vi "Pockels-Initialise sequence for funct acq.vi"() -> (1 "Count towards trigger target (ms)":dbl format="%#_9g", 2 "Excess (us)":dbl format="%#_9g", 3 "waveform out":waveform(dbl)(graph))   [LabVIEW 2017]
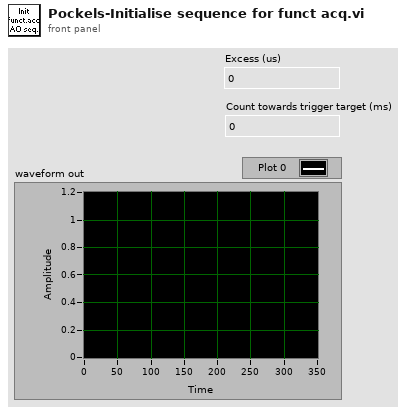
[diagram p1: front panel]
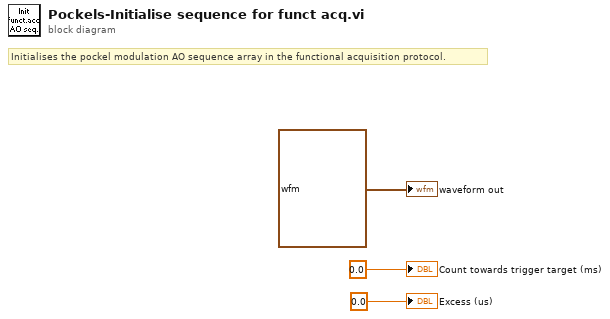
[diagram p0: block diagram]
diagram:
  # "Initialises the pockel modulation AO sequence array in the functional acquisition protocol."
  "waveform out" <- waveform(dbl) {"t0"=timestamp(0 s since 1904-01-01), "dt"=0.0, "Y"=[]} ("waveform out")
  "Excess (us)" <- 0.0 ("Count towards trigger target (us)")
  "Count towards trigger target (ms)" <- 0.0 ("Count towards trigger target (us)")
